vi "Read_WeldAutoParams_Local_ini.vi"(0 "TestCaseName_Config.ini File Path (Test case level)":path, 3 "error in":errorcluster) -> (5 "SC Parameters to BL (HEX format)":string, 6 "PC_AC Parameters to BL (HEX format)":string, 8 "[Initialization]":i32[](array[numeric]), 9 "[framework_settings]":string[](array[string]), 10 "error out":errorcluster)   [LabVIEW 2017]
uses:
  <vilib>/Utility/config.llb/Read Key (I32).vi
  <vilib>/Utility/config.llb/Read Key (String).vi
  Global_Variable_Status_Indicator.vi
  <vilib>/Utility/config.llb/Read Key (U32).vi
  <vilib>/Utility/config.llb/Read Key (Boolean).vi
  <vilib>/Utility/config.llb/NI_LVConfig.lvlib
panel:
  out "Size of PC_AC Parameters":u32
  out "Size of SC Parameters":u64
  # "READ WELD  AUTOMATION  PARAMETERS AND KEY VALUES"
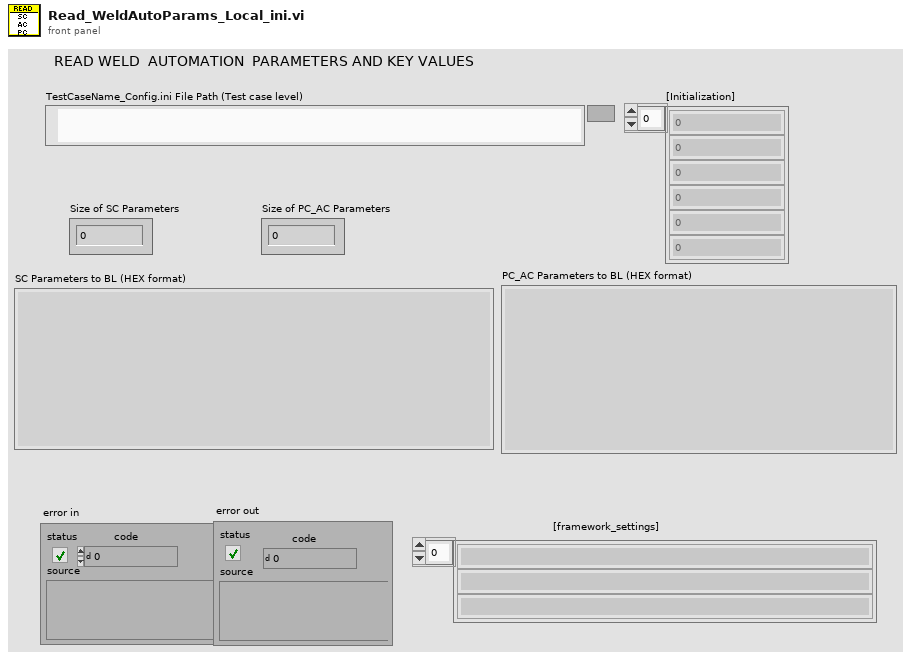
[diagram p1: front panel]
types:
  T1 = typedef "NI_LVConfig.lvlib/Config Data RefNum.ctl" = refnum<k1>
  T2 = enum16{"big-endian, network order", "native, host order", "little-endian"}
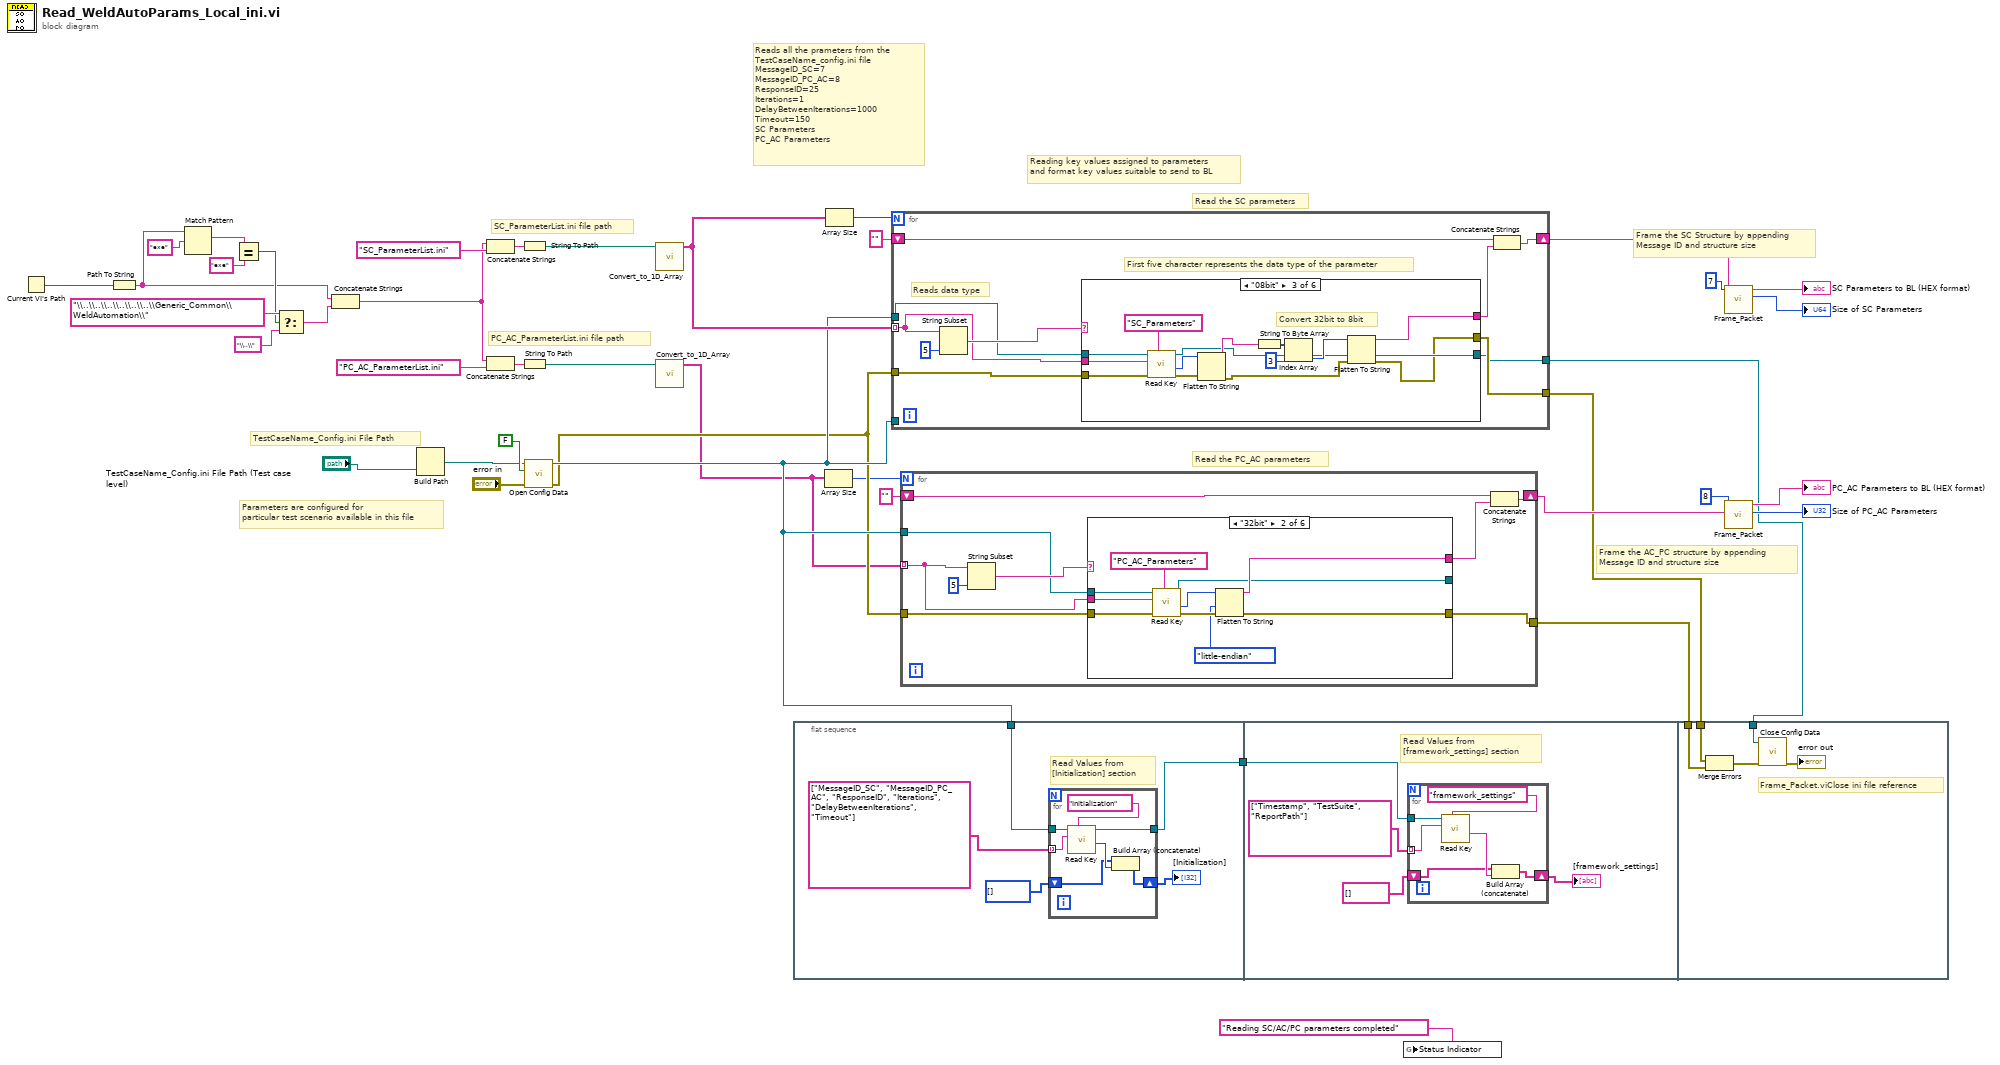
[diagram p0: block diagram]
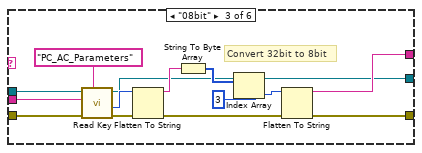
[diagram p3: hidden frame]
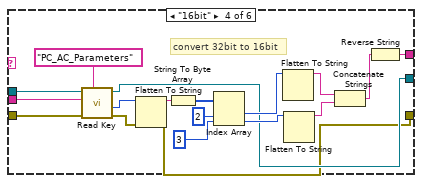
[diagram p4: hidden frame]
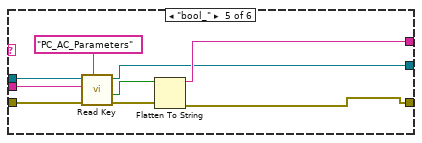
[diagram p5: hidden frame]
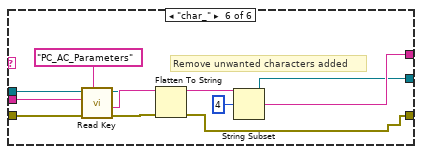
[diagram p6: hidden frame]
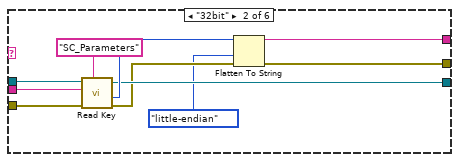
[diagram p8: hidden frame]
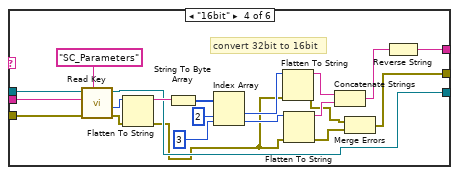
[diagram p9: hidden frame]
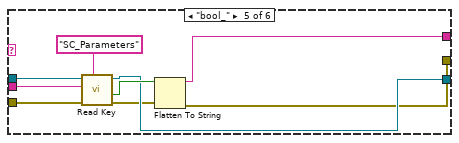
[diagram p10: hidden frame]
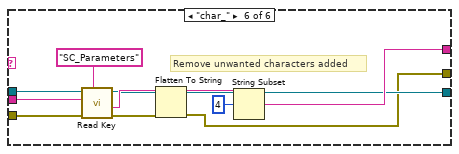
[diagram p11: hidden frame]
diagram:
  # "Frame the AC_PC structure by appending\nMessage ID and structure size"
  # "Frame the SC Structure by appending\nMessage ID and structure size"
  # "TestCaseName_Config.ini File Path"
  # "PC_AC_ParameterList.ini file path"
  # "SC_ParameterList.ini file path"
  # "Reads all the prameters from the \nTestCaseName_config.ini file\nMessageID_SC=7\nMessageID_PC_AC=8\nResponseID=25\nIterations=1\nDelayBetweenIterations=1000\nTimeout=150\nSC Parameters\nPC_AC Parameters"
  # "Read the SC parameters"
  # "Read the PC_AC parameters"
  # "Parameters are configured for \nparticular test scenario available in this file"
  # "Reading key values assigned to parameters\nand format key values suitable to send to BL"
  n1 = Current VI's Path() -> (path=w3:path)
  n2 = Path To String(path=w3) -> (string=w1:string)
  n3 = Match Pattern(string=w1, regular expression="exe") -> (match substring=w7:string)  [unwired: 1 in, 3 out]
  n4 = Equal?(x=w7, y="exe") -> (x = y?=w5:bool)
  n5 = Select(t="\\..\\..\\..\\..\\..\\..\\Generic_Common\\WeldAutomation\\" ("string"), s=w5, f="\\..\\" ("string")) -> (s? t:f=w8:string)
  n6 = Concatenate Strings(w1, w8) -> (w2:string)
  n7 = Build Path(name or relative path="TestCaseName_Config.ini File Path (Test case level)") -> (appended path=w40:path)  [unwired: 1 in]
  n8 = Concatenate Strings(w2, "SC_ParameterList.ini") -> (w29:string)
  n9 = Concatenate Strings(w2, "PC_AC_ParameterList.ini") -> (w28:string)
  n10 = String To Path(string=w29) -> (path=w27:path)
  n11 = String To Path(string=w28) -> (path=w22:path)
  n12 = call <vilib>:"Open Config Data.vi"("error in (no error)"="error in", "create file if necessary (T)"=FALSE ("create file if necessary? (T)"), "configuration file path"=w40) -> ("error out"=w33:errorcluster, "refnum"=w34:T1)  [unwired: 6 in, 1 out]
  n13 = call "Convert_to_1D_Array.vi"("Path"=w27) -> ("Array"=w38:string[])  [unwired: 10 in]
  n14 = call "Convert_to_1D_Array.vi"("Path"=w22) -> ("Array"=w23:string[])  [unwired: 10 in]
  n15 = flat-sequence {
    tunnel: w34 -> [w43]
    tunnel: [w42] -> w36
    tunnel: w36 -> [w54]
    tunnel: w15 -> [w66]
    tunnel: w14 -> [w65]
    tunnel: w13 -> [w64]
    frame #0 {
      # "Read Values from \n[Initialization] section"
      n16 = for {
        tunnel: string[] ["MessageID_SC", "MessageID_PC_AC", "ResponseID", "Iterations", "DelayBetweenIterations", "Timeout"] -> [w52] mode=indexing
        shift-right: [w53] -> w44
        shift-left: i32[] [] -> [w47]
        tunnel: w43 -> [w51]
        tunnel: [w50] -> w42
        n17 = call-poly <vilib>:"Read Key.vi"("section"="Initialization", "key"=w52, "refnum"=w51) -> ("value"=w48:i32, "refnum out"=w50:T1)  [unwired: 5 in, 2 out]
        n18 = Build Array (concatenate)(w47, w48) -> (w53:i32[])
      }
      "[Initialization]" <- w44
    }
    frame #1 {
      # "Read Values from \n[framework_settings] section"
      n19 = for {
        tunnel: string[] ["Timestamp", "TestSuite", "ReportPath"] -> [w63] mode=indexing
        shift-right: [w62] -> w57
        shift-left: string[] [] -> [w58]
        tunnel: w54 -> [w61]
        n20 = call-poly <vilib>:"Read Key.vi"("section"="framework_settings", "key"=w63, "refnum"=w61) -> ("value"=w59:string)  [unwired: 5 in, 3 out]
        n21 = Build Array (concatenate)(w58, w59) -> (w62:string[])
      }
      "[framework_settings]" <- w57
    }
    frame #2 {
      # "Frame_Packet.viClose ini file reference"
      n22 = Merge Errors(w66, w65) -> (w68:errorcluster)
      n23 = call <vilib>:"Close Config Data.vi"("error in (no error)"=w68, "refnum"=w64) -> ("error out"=→"error out":errorcluster)  [unwired: 8 in, 1 out]
    }
  }
  n24 = Array Size(array=w23) -> (size(s)=w11:i32)
  n25 = Array Size(array=w38) -> (size(s)=w12:i32)
  n26 = for {
    N: w12 -> [_]
    tunnel: w33 -> [w75]
    tunnel: w34 -> [w73]
    shift-right: [w76] -> w26
    shift-left: "" -> [w77]
    tunnel: w38 -> [w72] mode=indexing
    tunnel: w34 -> [_]
    tunnel: [w70] -> w15
    tunnel: [w69] -> w13
    # "First five character represents the data type of the parameter"
    # "Reads data type"
    n27 = String Subset(string=w72, length (rest)=5 ("length (rest)")) -> (substring=w74:string)  [unwired: 1 in]
    n28 = case shown="\"08bit\"" w74 {
      tunnel: w75 -> [w80 w90 w104 w125 w134 w145]
      tunnel: w73 -> [w79 w89 w103 w124 w133 w144]
      tunnel: w72 -> [_ w87 w101 w122 w131 w142]
      tunnel: [_ w85 w95 w106 w129 w138] -> w71
      tunnel: [w79 w84 w94 w112 w128 w137] -> w69
      tunnel: [w80 w82 w91 w107 w126 w135] -> w70
      frame Default {
      }
      frame "32bit" {
        n29 = call-poly <vilib>:"Read Key.vi"("section"="SC_Parameters", "error in (no error)"=w90, "key"=w87, "refnum"=w89) -> ("error out"=w83:errorcluster, "value"=w86:u32, "refnum out"=w84:T1)  [unwired: 1 in, 4 out]
        n30 = Flatten To String(anything=w86, byte order (0:big-endian, network order)=T2."little-endian", error in (no error)=w83) -> (data string=w85:string, error out=w82:errorcluster)  [unwired: 1 in, 1 out]
      }
      frame "08bit" {
        # "Convert 32bit to 8bit"
        n31 = call-poly <vilib>:"Read Key.vi"("section"="SC_Parameters", "error in (no error)"=w104, "key"=w101, "refnum"=w103) -> ("error out"=w93:errorcluster, "value"=w100:u32, "refnum out"=w94:T1)  [unwired: 1 in, 4 out]
        n32 = Flatten To String(anything=w100, error in (no error)=w93) -> (data string=w99:string, error out=w92:errorcluster)  [unwired: 2 in, 1 out]
        n33 = String To Byte Array(string=w99) -> (unsigned byte array=w98:u8[])
        n34 = Index Array(array=w98, index=3) -> (element=w96:u8)
        n35 = Flatten To String(anything=w96, error in (no error)=w92) -> (data string=w95:string, error out=w91:errorcluster)  [unwired: 2 in, 1 out]
      }
      frame "16bit" {
        # "convert 32bit to 16bit"
        n36 = call-poly <vilib>:"Read Key.vi"("section"="SC_Parameters", "error in (no error)"=w125, "key"=w122, "refnum"=w124) -> ("error out"=w111:errorcluster, "value"=w121:u32, "refnum out"=w112:T1)  [unwired: 1 in, 4 out]
        n37 = Flatten To String(anything=w121, error in (no error)=w111) -> (data string=w120:string, error out=w110:errorcluster)  [unwired: 2 in, 1 out]
        n38 = String To Byte Array(string=w120) -> (unsigned byte array=w119:u8[])
        n39 = Index Array(array=w119, index #1=2 ("index"), index #2=3 ("index")) -> (element #1=w115:u8, element #2=w114:u8)
        n40 = Flatten To String(anything=w115, error in (no error)=w110) -> (data string=w113:string, error out=w109:errorcluster)  [unwired: 2 in, 1 out]
        n41 = Flatten To String(anything=w114, error in (no error)=w110) -> (data string=w116:string, error out=w108:errorcluster)  [unwired: 2 in, 1 out]
        n42 = Concatenate Strings(w113, w116) -> (w105:string)
        n43 = Merge Errors(w109, w108) -> (w107:errorcluster)
        n44 = Reverse String(1:w105) -> (0:w106:string)
      }
      frame "bool_" {
        n45 = call-poly <vilib>:"Read Key.vi"("section"="SC_Parameters", "error in (no error)"=w134, "key"=w131, "refnum"=w133) -> ("error out"=w127:errorcluster, "value"=w130:bool, "refnum out"=w128:T1)  [unwired: 1 in, 4 out]
        n46 = Flatten To String(anything=w130, error in (no error)=w127) -> (data string=w129:string, error out=w126:errorcluster)  [unwired: 2 in, 1 out]
      }
      frame "char_" {
        # "Remove unwanted characters added"
        n47 = call-poly <vilib>:"Read Key.vi"("section"="SC_Parameters", "error in (no error)"=w145, "key"=w142, "refnum"=w144) -> ("error out"=w136:errorcluster, "value"=w141:string, "refnum out"=w137:T1)  [unwired: 2 in, 3 out]
        n48 = Flatten To String(anything=w141, error in (no error)=w136) -> (data string=w140:string, error out=w135:errorcluster)  [unwired: 2 in, 1 out]
        n49 = String Subset(string=w140, offset (0)=4) -> (substring=w138:string)  [unwired: 1 in]
      }
    }
    n50 = Concatenate Strings(w77, w71) -> (w76:string)
  }
  n51 = for {
    N: w11 -> [_]
    tunnel: w23 -> [w151] mode=indexing
    tunnel: w34 -> [w152]
    tunnel: w33 -> [w150]
    shift-right: [w147] -> w18
    shift-left: "" -> [w149]
    tunnel: [w146] -> w14
    n52 = String Subset(string=w151, length (rest)=5 ("length (rest)")) -> (substring=w153:string)  [unwired: 1 in]
    n53 = case shown="\"32bit\"" w153 {
      tunnel: w150 -> [w155 w166 w180 w198 w207 w218]
      tunnel: w152 -> [w156 w165 w179 w197 w206 w217]
      tunnel: w151 -> [_ w163 w177 w195 w204 w215]
      tunnel: [_ w161 w171 w182 w202 w211] -> w148
      tunnel: [w156 w160 w170 w185 w201 w210] -> _
      tunnel: [w155 w158 w167 w183 w199 w208] -> w146
      frame Default {
      }
      frame "32bit" {
        n54 = call-poly <vilib>:"Read Key.vi"("section"="PC_AC_Parameters", "error in (no error)"=w166, "key"=w163, "refnum"=w165) -> ("error out"=w159:errorcluster, "value"=w162:u32, "refnum out"=w160:T1)  [unwired: 1 in, 4 out]
        n55 = Flatten To String(anything=w162, byte order (0:big-endian, network order)=T2."little-endian", error in (no error)=w159) -> (data string=w161:string, error out=w158:errorcluster)  [unwired: 1 in, 1 out]
      }
      frame "08bit" {
        # "Convert 32bit to 8bit"
        n56 = call-poly <vilib>:"Read Key.vi"("section"="PC_AC_Parameters", "error in (no error)"=w180, "key"=w177, "refnum"=w179) -> ("error out"=w169:errorcluster, "value"=w176:u32, "refnum out"=w170:T1)  [unwired: 1 in, 4 out]
        n57 = Flatten To String(anything=w176, error in (no error)=w169) -> (data string=w175:string, error out=w168:errorcluster)  [unwired: 2 in, 1 out]
        n58 = String To Byte Array(string=w175) -> (unsigned byte array=w174:u8[])
        n59 = Index Array(array=w174, index=3) -> (element=w172:u8)
        n60 = Flatten To String(anything=w172, error in (no error)=w168) -> (data string=w171:string, error out=w167:errorcluster)  [unwired: 2 in, 1 out]
      }
      frame "16bit" {
        # "convert 32bit to 16bit"
        n61 = call-poly <vilib>:"Read Key.vi"("section"="PC_AC_Parameters", "error in (no error)"=w198, "key"=w195, "refnum"=w197) -> ("error out"=w184:errorcluster, "value"=w194:u32, "refnum out"=w185:T1)  [unwired: 1 in, 4 out]
        n62 = Flatten To String(anything=w194, error in (no error)=w184) -> (data string=w193:string, error out=w183:errorcluster)  [unwired: 2 in, 1 out]
        n63 = String To Byte Array(string=w193) -> (unsigned byte array=w192:u8[])
        n64 = Index Array(array=w192, index #1=2 ("index"), index #2=3 ("index")) -> (element #1=w188:u8, element #2=w187:u8)
        n65 = Flatten To String(anything=w188) -> (data string=w186:string)  [unwired: 3 in, 2 out]
        n66 = Flatten To String(anything=w187) -> (data string=w189:string)  [unwired: 3 in, 2 out]
        n67 = Concatenate Strings(w186, w189) -> (w181:string)
        n68 = Reverse String(1:w181) -> (0:w182:string)
      }
      frame "bool_" {
        n69 = call-poly <vilib>:"Read Key.vi"("section"="PC_AC_Parameters", "error in (no error)"=w207, "key"=w204, "refnum"=w206) -> ("error out"=w200:errorcluster, "value"=w203:bool, "refnum out"=w201:T1)  [unwired: 1 in, 4 out]
        n70 = Flatten To String(anything=w203, error in (no error)=w200) -> (data string=w202:string, error out=w199:errorcluster)  [unwired: 2 in, 1 out]
      }
      frame "char_" {
        # "Remove unwanted characters added"
        n71 = call-poly <vilib>:"Read Key.vi"("section"="PC_AC_Parameters", "error in (no error)"=w218, "key"=w215, "refnum"=w217) -> ("error out"=w209:errorcluster, "value"=w214:string, "refnum out"=w210:T1)  [unwired: 2 in, 3 out]
        n72 = Flatten To String(anything=w214, error in (no error)=w209) -> (data string=w213:string, error out=w208:errorcluster)  [unwired: 2 in, 1 out]
        n73 = String Subset(string=w213, offset (0)=4) -> (substring=w211:string)  [unwired: 1 in]
      }
    }
    n74 = Concatenate Strings(w149, w148) -> (w147:string)
  }
  n75 = global write "Global_Variable_Status_Indicator.vi" "Status Indicator"("Reading SC/AC/PC parameters completed") -> ()
  n76 = call "Frame_Packet.vi"("String in"=w26, "Numeric in"=u32 7) -> ("Numeric out"=→"Size of SC Parameters":i32, "String out"=→"SC Parameters to BL (HEX format)":string)  [unwired: 8 in]
  n77 = call "Frame_Packet.vi"("String in"=w18, "Numeric in"=u32 8) -> ("Numeric out"=→"Size of PC_AC Parameters":i32, "String out"=→"PC_AC Parameters to BL (HEX format)":string)  [unwired: 8 in]
